vi "Page_Exclusions_ReadShared.vi"(8 "error in (no error)":errorcluster, 10 "ctlReferences":T1, 11 "AB_Application in":refnum<class "AB_Application.lvclass">) -> (0 "error out":errorcluster, 3 "AB_Application out":refnum<class "AB_Application.lvclass">)   [LabVIEW 2020, in "AB_Application.lvclass"]
uses:
  <vilib>/AppBuilder/AB_Classes/Application/AB_Application.lvclass
  <vilib>/AppBuilder/AB_Classes/Application/AB_Application.lvclass/AB_Application.ctl
  <resource>/Framework/Providers/Builds/AppBuilder/AB_UI_Page_Exclusions_References.ctl
panel:
  in  "Web services warning":bool
  in  "Library file":bool
  in  "Library members":bool
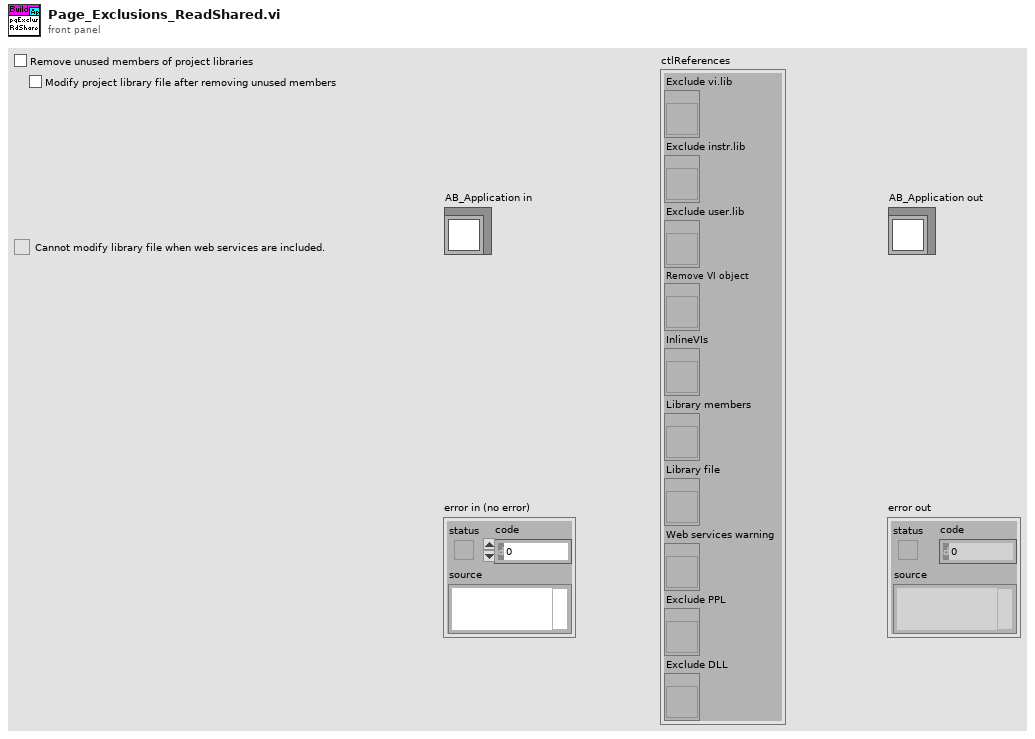
[diagram p1: front panel]
types:
  T1 = typedef "AB_UI_Page_Exclusions_References.ctl" = cluster{"Exclude vi.lib":refnum<vi>, "Exclude instr.lib":refnum<vi>, "Exclude user.lib":refnum<vi>, "Remove VI object":refnum<vi>, "InlineVIs":refnum<vi>, "Library members":refnum<vi>, "Library file":refnum<vi>, "Web services warning":refnum<vi>, "Exclude PPL":refnum<vi>, "Exclude DLL":refnum<vi>}
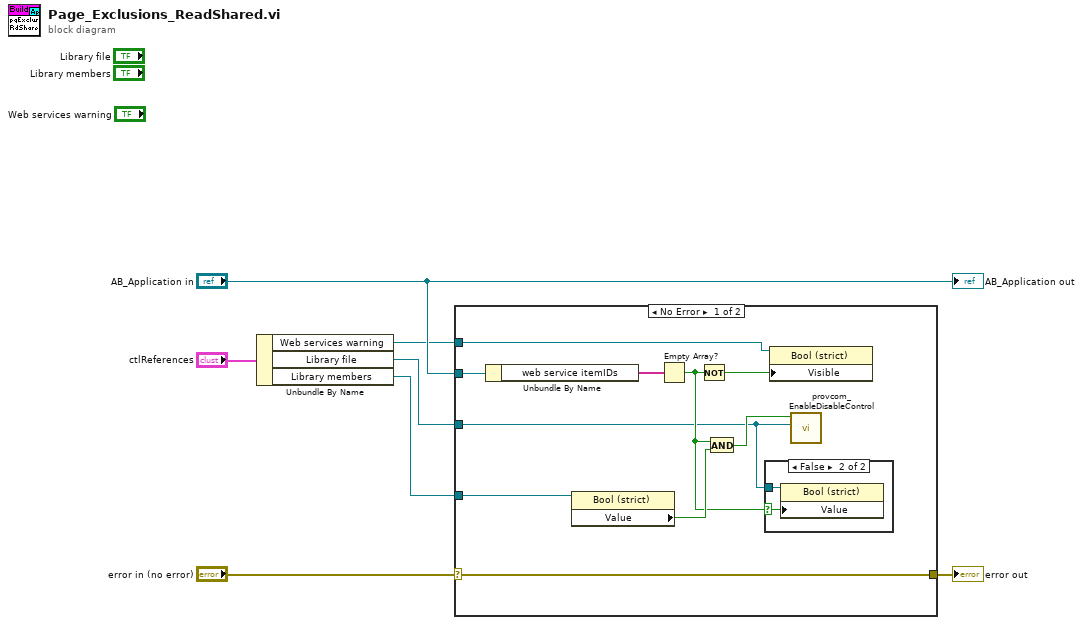
[diagram p0: block diagram]
diagram:
  n1 = Unbundle By Name("ctlReferences") -> ("Web services warning"=w3:refnum<vi>, "Library file"=w2:refnum<vi>, "Library members"=w1:refnum<vi>)
  n2 = case shown="No Error" "error in (no error)" {
    selector: "error in (no error)" -> [w8 w20]
    tunnel: "AB_Application in" -> [w12 _]
    tunnel: w2 -> [w11 _]
    tunnel: w1 -> [w10 _]
    tunnel: w3 -> [w9 _]
    tunnel: [w8 w20] -> w5
    frame No Error {
      n3 = Unbundle By Name(w12) -> ("web service itemIDs"=w16:string[])
      n4 = property class="Bool (strict)"(reference=w10) -> ("Value"=w15:bool)  [unwired: 1 in, 2 out]
      n5 = Empty Array?(array=w16) -> (empty?=w13:bool)
      n6 = Not(x=w13) -> (.not. x?=w17:bool)
      n7 = And(x=w13, y=w15) -> (x .and. y?=w14:bool)
      n8 = case shown="False" w13 {
        selector: w13 -> [_ w18]
        tunnel: w11 -> [_ w19]
        frame True {
        }
        frame False {
          n9 = property class="Bool (strict)"(reference=w19, "Value"=w18) -> ()  [unwired: 1 in, 2 out]
        }
      }
      n10 = property class="Bool (strict)"(reference=w9, "Visible"=w17) -> ()  [unwired: 1 in, 2 out]
      n11 = call <resource>:"provcom_EnableDisableControl.vi"("Control"=w11, "Enable (TRUE)"=w14) -> ()  [unwired: 9 in, 1 out]
    }
    frame Error {
    }
  }
  "error out" <- w5
  "AB_Application out" <- "AB_Application in"
